vi "DP Panel.vi"() -> ()   [LabVIEW 2014]
uses:
  Control go.ctl
  <vilib>/Utility/miscctls.llb/LVCursorListTypeDef.ctl
  <vilib>/imath/engines/lvmath2/RunTimeEngine/IndexRead/NIMS V(S).vi
  <instcachedir>/0/NIMS V(S)_0488751826AF41519A22953C041130DC.lvgen/NIMS V(S)_0488751826AF41519A22953C041130DC_000.vi
  <vilib>/imathl/engines/lvmath/Functions/Error Handling/Create Error.vi
  <vilib>/imath/engines/lvmath2/RunTimeEngine/NodeEndStatement/NIMS_NodeEndStatement_Output.vi
  <instcachedir>/0/NIMS_NodeEndStatement_Output_53EC0D466D134D7ABD903AC30B43404B.lvgen/NIMS_NodeEndStatement_Output_53EC0D466D134D7ABD903AC30B43404B_001.vi
  <vilib>/imath/engines/lvmath2/RunTimeEngine/ErrorHandling/NIMS_Finalize Error.vi
panel:
  in  "Break":bool
  in  "max [deg/s]":dbl=10.0
  in  "v_max":dbl=0.3 caption="max vel [m/s]"
  in  "Depth Limit":dbl=5.0
  out "Dynamic Positioning Help":string
  in  "Cursor List":T1
  in  "Eta":dbl[](array[numeric])
  in  "TCPConRef":refnum<k5>
  out "String 4":string
  out "String 3":string
  out "String 2":string
  out "String":string
  in  "Heading":dbl
  in  "Depth":dbl
  in  "East":dbl format="%#.2f"
  in  "North":dbl format="%#.2f"
  in  "Mode Selection":string(combo)
  in  "Make Change":T2
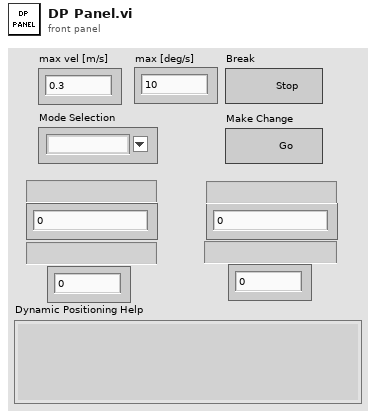
[diagram p1: front panel]
types:
  T1 = typedef "LVCursorListTypeDef.ctl" = cluster{"Name":string, "Color":u32, "Style":u8, "Point Style":u8, "Name Visible":bool, "Allow Drag":bool, "Cursor Mode":u32, "Plot":i32, "Index":i32, "Position":cluster{"X":dbl, "Y":dbl}, "X Scale":u32, "Y Scale":u32, "Watch Plots":i32[], "Watch All Plots":bool, "Plot Area":i32, "Label Offset":cluster{"X":dbl, "Y":dbl}}[]
  T2 = typedef "Control go.ctl" = bool
  T3 = cluster{"Name":string, "Color":u32, "Style":u8, "Point Style":u8, "Name Visible":bool, "Allow Drag":bool, "Cursor Mode":u32, "Plot":i32, "Index":i32, "Position":cluster{"X":dbl, "Y":dbl}, "X Scale":u32, "Y Scale":u32, "Watch Plots":i32[], "Watch All Plots":bool, "Plot Area":i32, "Label Offset":cluster{"X":dbl, "Y":dbl}}
  T4 = cluster{"Name":string, "Color":u32, "Style":u8, "Point Style":u8, "Name Visible":bool, "Allow Drag":bool, "Cursor Mode":u32, "Plot":i32, "Index":i32, "Position":cluster{"X":dbl, "Y":dbl}, "X Scale":u32, "Y Scale":u32, "Watch Plots":i32[], "Watch All Plots":bool, "Plot Area":i32, "Label Offset":cluster{"X":dbl, "Y":dbl}}[]
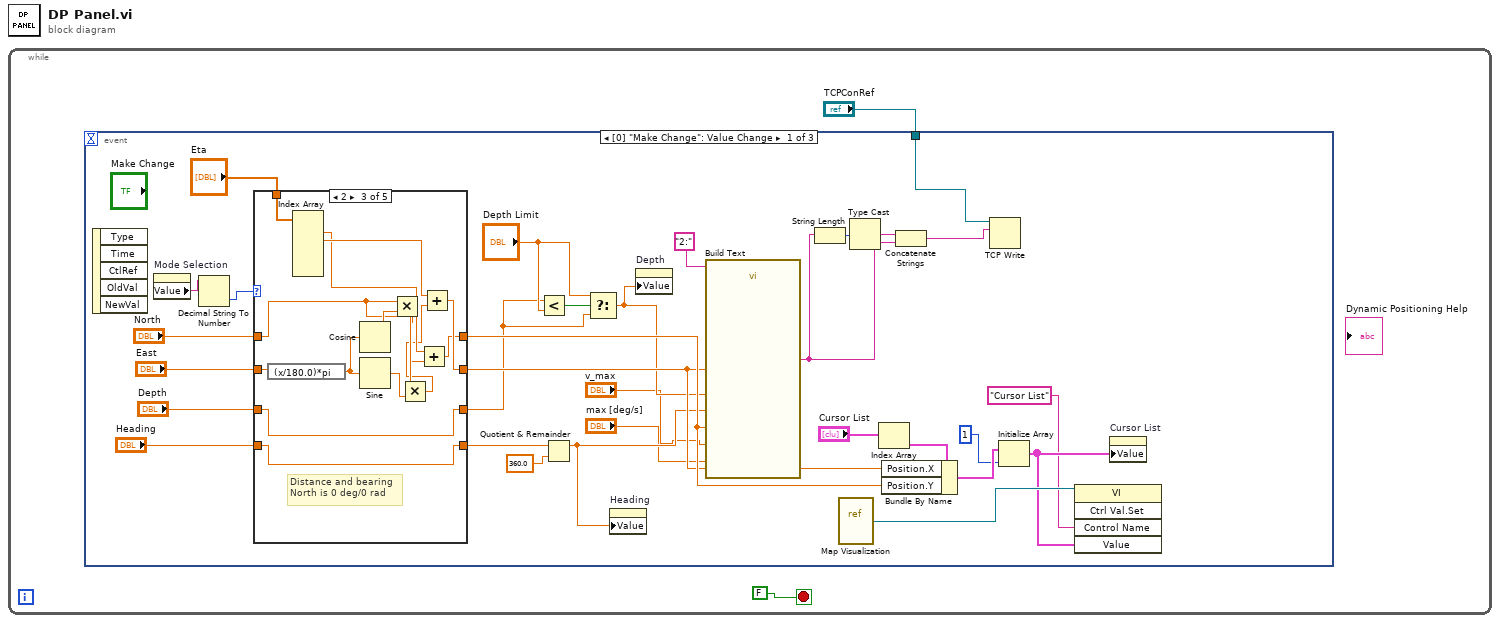
[diagram p0: block diagram]
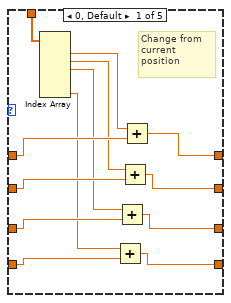
[diagram p2: hidden frame]
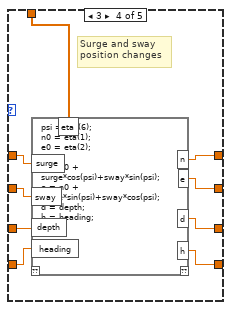
[diagram p4: hidden frame]
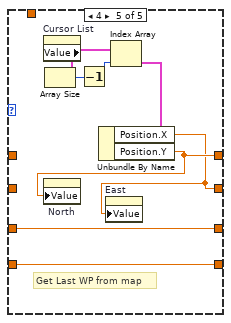
[diagram p5: hidden frame]
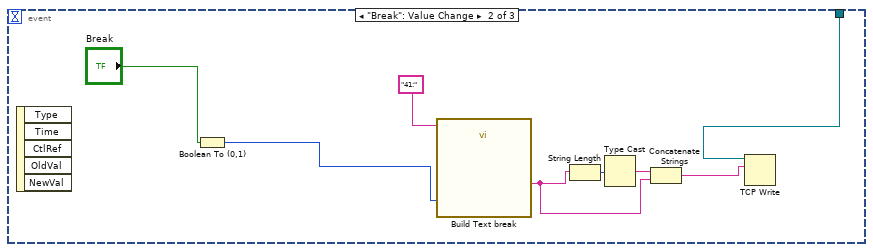
[diagram p6: hidden frame]
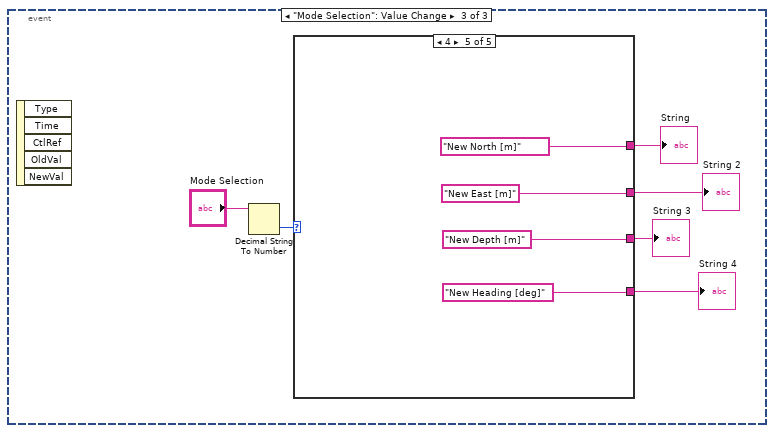
[diagram p7: hidden frame]
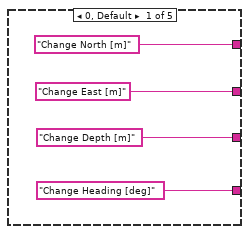
[diagram p8: hidden frame]
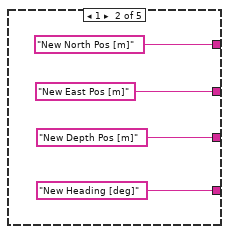
[diagram p9: hidden frame]
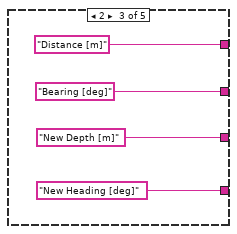
[diagram p10: hidden frame]
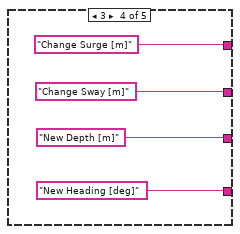
[diagram p11: hidden frame]
diagram:
  n1 = while {
    stop <- FALSE stop-if-true
    n2 = event shown="[0] \"Make Change\": Value Change" {
      selector: _ -> [_ _ _]
      dyn-events: _ -> [_ _ _]
      timeout: _ -> [_ _ _]
      tunnel: "TCPConRef" -> [w3 w203 _]
      event Value Change {
        n3 = event-data() -> ()  [unwired: 1 in, 5 out]
        n4 = property on="Mode Selection" class="CmbBox"() -> ("Value"=w31:string)  [unwired: 2 in, 2 out]
        n5 = Decimal String To Number(string=w31) -> (number=w27:i32)  [unwired: 2 in, 1 out]
        n6 = case shown="2" w27 {
          tunnel: "North" -> [w44 w50 w60 w68 _]
          tunnel: "East" -> [w40 w49 w64 w67 _]
          tunnel: "Depth" -> [w41 w48 w52 w66 w202]
          tunnel: "Heading" -> [w42 w47 w51 w65 w201]
          tunnel: [w43 w50 w55 w72 w196] -> w14
          tunnel: [w39 w49 w57 w71 w195] -> w13
          tunnel: [w38 w48 w52 w70 w202] -> w7
          tunnel: [w37 w47 w51 w69 w201] -> w15
          tunnel: "Eta" -> [w46 _ w59 w73 _]
          frame 0, Default {
            # "Change from \ncurrent \nposition"
            n7 = Index Array(array=w46) -> (element #1=w45:dbl, element #2=w36:dbl, element #3=w35:dbl, element #6=w34:dbl)  [unwired: 6 in, 2 out]
            n8 = Add(x=w34, y=w42) -> (x+y=w37:dbl)
            n9 = Add(x=w35, y=w41) -> (x+y=w38:dbl)
            n10 = Add(x=w36, y=w40) -> (x+y=w39:dbl)
            n11 = Add(x=w45, y=w44) -> (x+y=w43:dbl)
          }
          frame 1 {
            # "New Position"
          }
          frame 2 {
            # "Distance and bearing\nNorth is 0 deg/0 rad"
            n12 = expression code="(x/180.0)*pi" ("degrees to radians")(w64) -> (w63:dbl)
            n13 = Index Array(array=w59) -> (element #1=w56:dbl, element #2=w58:dbl)  [unwired: 6 in, 4 out]
            n14 = Cosine(x=w63) -> (cos(x)=w62:dbl)
            n15 = Sine(x=w63) -> (sin(x)=w61:dbl)
            n16 = Multiply(x=w60, y=w62) -> (x*y=w54:dbl)
            n17 = Multiply(x=w60, y=w61) -> (x*y=w53:dbl)
            n18 = Add(x=w56, y=w54) -> (x+y=w55:dbl)
            n19 = Add(x=w58, y=w53) -> (x+y=w57:dbl)
          }
          frame 3 {
            # "Surge and sway\nposition changes"
            n20 = mathscript code="psi = eta(6);\nn0 = eta(1);\ne0 = eta(2);\n\nn = n0 + surge*cos(psi)+sway*sin(psi);\ne = n0 + surge*sin(psi)+sway*cos(psi);\nd = depth;\nh = heading;"("eta"=w73, "surge"=w68, "sway"=w67, "depth"=w66, "heading"=w65) -> ("n"=w72:dbl, "e"=w71:dbl, "d"=w70:dbl, "h"=w69:dbl)  [unwired: 1 in, 1 out]
          }
          frame 4 {
            # "Get Last WP from map"
            n21 = property on="Cursor List" class="Arr (strict)"() -> ("Value"=w200:T1)  [unwired: 2 in, 2 out]
            n22 = Array Size(array=w200) -> (size(s)=w199:i32)
            n23 = Decrement(x=w199) -> (x-1=w198:i32)
            n24 = Index Array(array=w200, index=w198) -> (element=w197:T3)
            n25 = Unbundle By Name(w197) -> ("Position.X"=w195:dbl, "Position.Y"=w196:dbl)
            n26 = property on="North" class="DigNum (strict)"("Value"=w196) -> ()  [unwired: 2 in, 2 out]
            n27 = property on="East" class="DigNum (strict)"("Value"=w195) -> ()  [unwired: 2 in, 2 out]
          }
        }
        n28 = Less?(x=w7, y="Depth Limit") -> (x < y?=w9:bool)
        n29 = Quotient & Remainder(x=w15, y=360.0) -> (x-y*floor(x/y)=w11:dbl)  [unwired: 1 out]
        n30 = Select(t="Depth Limit", s=w9, f=w7) -> (s? t:f=w6:dbl)
        n31 = property on="Heading" class="DigNum (strict)"("Value"=w11) -> ()  [unwired: 2 in, 2 out]
        n32 = property on="Depth" class="DigNum (strict)"("Value"=w6) -> ()  [unwired: 2 in, 2 out]
        n33 = call "Build Text"("Beginning Text"="2:", "Heading"=w11, "r_max"="max [deg/s]", "North"=w14, "East"=w13, "Depth"=w6, "v_max"="v_max") -> ("Result"=w29:string)  [unwired: 7 in, 1 out]
        n34 = String Length(string=w29) -> (length=w33:i32)
        n35 = vi-ref "Map Visualization.vi"() -> (w19:refnum<vi>)
        n36 = Type Cast(x=w33) -> (*(type *) &x=w32:string)  [unwired: 1 in]
        n37 = Index Array(array="Cursor List") -> (element=w21:T3)  [unwired: 1 in]
        n38 = Bundle By Name(cluster=w21, "Position.X"=w13, "Position.Y"=w14) -> (w20:T3)
        n39 = Concatenate Strings(w32, w29) -> (w28:string)
        n40 = TCP Write(connection ID=w3, data in=w28) -> ()  [unwired: 2 in, 3 out]
        n41 = Initialize Array(w20, 1) -> (w18:T4)
        n42 = invoke class="VI" method="Ctrl Val.Set"(reference=w19, "Control Name"="Cursor List", "Value"=w18) -> ()  [unwired: 2 in, 5 out]
        n43 = property on="Cursor List" class="Arr (strict)"("Value"=w18) -> ()  [unwired: 2 in, 2 out]
      }
      event "Break": Value Change {
        n44 = event-data() -> ()  [unwired: 1 in, 5 out]
        n45 = Boolean To (0,1)(Boolean="Break") -> (0, 1=w204:i16)
        n46 = call "Build Text break"("Beginning Text"="41:", "break"=w204) -> ("Result"=w206:string)  [unwired: 12 in, 1 out]
        n47 = String Length(string=w206) -> (length=w208:i32)
        n48 = Type Cast(x=w208) -> (*(type *) &x=w209:string)  [unwired: 1 in]
        n49 = Concatenate Strings(w209, w206) -> (w210:string)
        n50 = TCP Write(connection ID=w203, data in=w210) -> ()  [unwired: 2 in, 3 out]
      }
      event "Mode Selection": Value Change {
        n51 = event-data() -> ()  [unwired: 1 in, 5 out]
        n52 = Decimal String To Number(string="Mode Selection") -> (number=w216:i32)  [unwired: 2 in, 1 out]
        n53 = case shown="4" w216 {
          tunnel: ["Change North [m]" "New North Pos [m]" "Distance [m]" "Change Surge [m]" "New North [m]"] -> w214
          tunnel: ["Change East [m]" "New East Pos [m]" "Bearing [deg]" "Change Sway [m]" "New East [m]"] -> w213
          tunnel: ["Change Depth [m]" "New Depth Pos [m]" "New Depth [m]" "New Depth [m]" "New Depth [m]"] -> w212
          tunnel: ["Change Heading [deg]" "New Heading [deg]" "New Heading [deg]" "New Heading [deg]" "New Heading [deg]"] -> w211
          frame 0, Default {
          }
          frame 1 {
          }
          frame 2 {
          }
          frame 3 {
          }
          frame 4 {
          }
        }
        "String" <- w214
        "String 2" <- w213
        "String 3" <- w212
        "String 4" <- w211
      }
    }
  }
